vi "Get Data.vi"(8 "error in":errorcluster, 11 "nPAS in":refnum<class "nPAS.lvclass">) -> (0 "error out":errorcluster, 3 "nPAS out":refnum<class "nPAS.lvclass">)   [LabVIEW 2018, in "gPAS Library.lvlib" / "nPAS.lvclass"]
doc: "Here you will do all of your acquisition. The acquisition is going to be implementation dependent, but at the bare minimum the class which inherits the PAS will have to retrieve the speaker signal(s). The data that is acquired in this cycle will be piped to the <b>Analyze Data</b> VI in the next cycle."
uses:
  nPAS.lvclass
  C:/Program Files (x86)/National Instruments/LabVIEW 2018/vi.lib/MSR Consulting, LLC/General Reuse/Instrument/Instrument.lvclass
  <vilib>/MSR Consulting, LLC/General Reuse/PAS/Data/Main/PAS Data.lvclass
  C:/Program Files (x86)/National Instruments/LabVIEW 2018/vi.lib/MSR Consulting, LLC/General Reuse/Data/Data.lvclass
  <vilib>/MSR Consulting, LLC/General Reuse/Instrument/Instrument.lvclass/Instrument.ctl
  <vilib>/MSR Consulting, LLC/General Reuse/PAS/Data/Cell/PAS Cell Data.lvclass/PAS Cell Data.ctl
  <vilib>/MSR Consulting, LLC/General Reuse/Instrument/Read Data.vi
  <vilib>/MSR Consulting, LLC/General Reuse/PAS/Data/Cell/Write lRMS.vi
  <vilib>/MSR Consulting, LLC/General Reuse/Instrument/Write Data.vi
  <vilib>/MSR Consulting, LLC/General Reuse/Instrument/Read Log Session.vi
  <vilib>/MSR Consulting, LLC/General Reuse/PAS/Data/Cell/PAS Cell Data.lvclass
  <vilib>/Utility/error.llb/Error Cluster From Error Code.vi
  <vilib>/rvi/errors/niLvFpgaAdjustHostInterfaceError.vi
  <vilib>/MSR Consulting, LLC/General Reuse/PAS/Data/Main/Read CellData.vi
  <vilib>/MSR Consulting, LLC/General Reuse/Data/Write measTime.vi
  <vilib>/MSR Consulting, LLC/General Reuse/PAS/Data/Cell/Write timeData.vi
  <vilib>/MSR Consulting, LLC/General Reuse/PAS/Data/Cell/Write lasDiodeData.vi
  <vilib>/MSR Consulting, LLC/General Reuse/PAS/Data/Main/Write CellData.vi
  <vilib>/rvi/interface/nirviMethod/nirviMethod.xnode
  FPGA Ref.ctl
  FPGA Bitfiles/server.lvbitx
  <vilib>/rvi/interface/nirviReadWriteControl/nirviReadWriteControl.xnode
  <vilib>/MSR Consulting, LLC/General Reuse/Data/Data.lvclass
  <vilib>/MSR Consulting, LLC/General Reuse/Session APIs/_Session Fwk/Session - Root.lvclass
  <vilib>/MSR Consulting, LLC/General Reuse/Session APIs/Session Log/System Log.lvclass
  <vilib>/FPGAPlugInAG/cRIO-9081/niLvFpga_ReadFifo_cRIO-9081.vi
  <vilib>/rvi/errors/niLvFpgaMergeErrorWithErrorCode.vi
  NiFpgaLv.dll
panel:
  out "Elements Remaining":u32
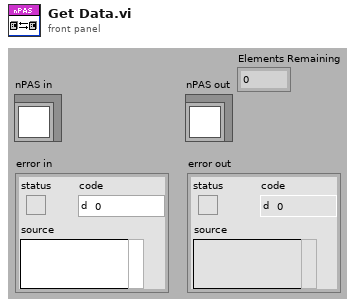
[diagram p1: front panel]
types:
  T1 = typedef "FPGA Ref.ctl" = refnum<k20>
  T2 = typedef "Session - Root.lvclass/Session Handle.ctl" = refnum<data-value>
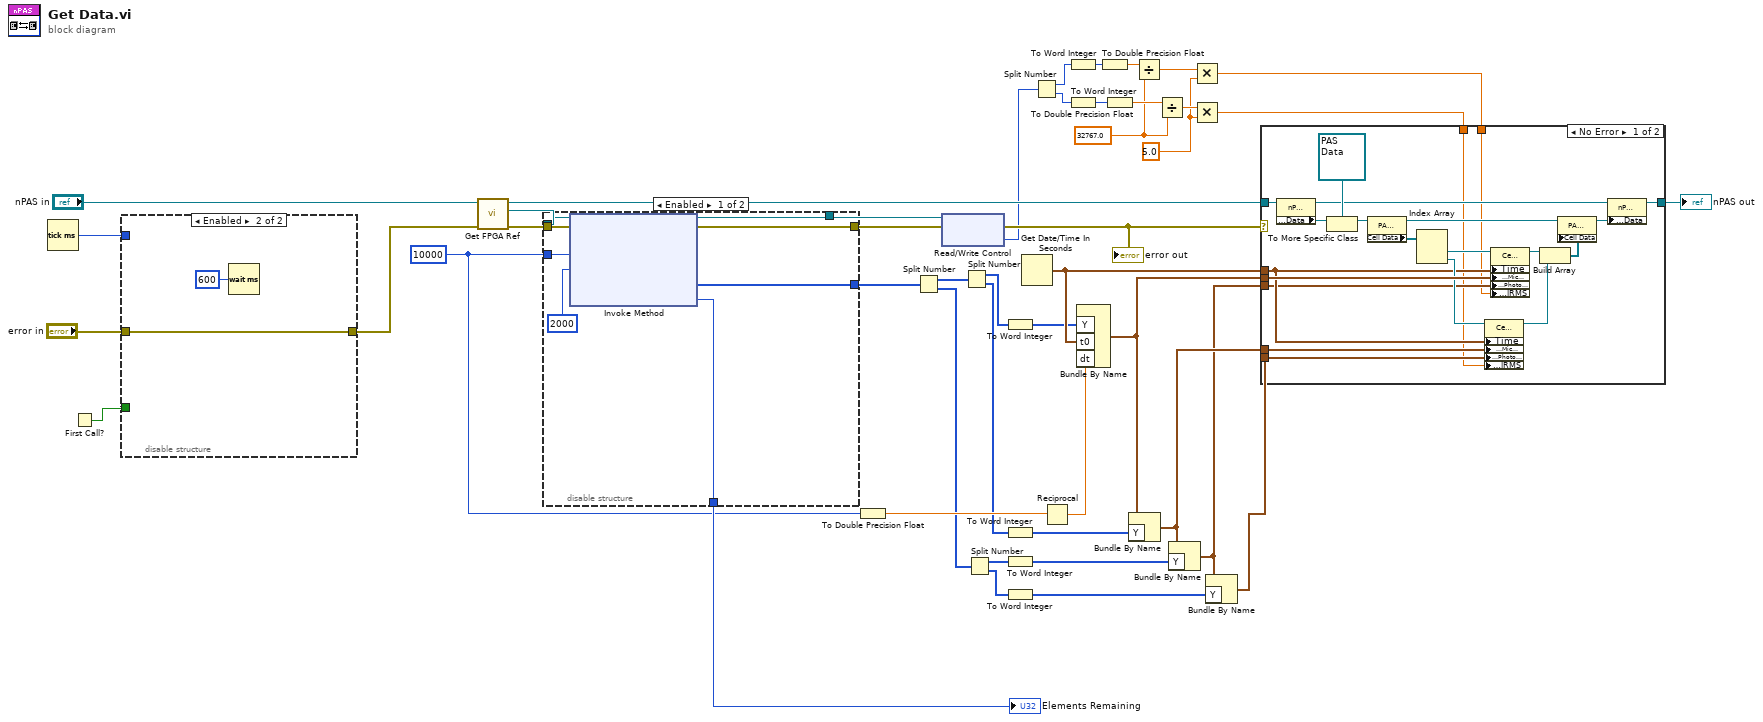
[diagram p0: block diagram]
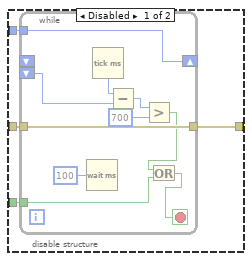
[diagram p2: hidden frame]
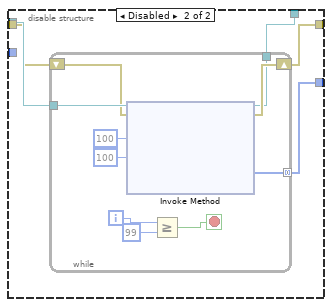
[diagram p3: hidden frame]
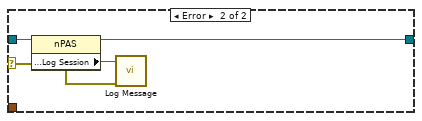
[diagram p4: hidden frame]
diagram:
  w7 = 5.0 ("y")
  w10 = 32767.0
  w42 = u32 10000 ("Number of Elements")
  n1 = Tick Count (ms)() -> (millisecond timer value=w2:u32)
  n2 = First Call?() -> (First Call?: T/F=w1:bool)
  n3 = disable-structure shown="Enabled" {
    disable-tunnel: "error in" -> [w49 w60]
    disable-tunnel: [w48 w60] -> w3
    disable-tunnel: w2 -> [w47 _]
    disable-tunnel: w1 -> [w46 _]
    frame Disabled {
      n4 = while {
        tunnel: w49 -> [w58]
        tunnel: [w58] -> w48
        tunnel: w47 -> [w57]
        shift-right: [w57] -> _
        shift-left: _ -> [_]
        shift-left: _ -> [w55]
        tunnel: w46 -> [w51]
        stop <- w50 stop-if-true
        n5 = Wait (ms)(milliseconds to wait=u32 100) -> ()  [unwired: 1 out]
        n6 = Tick Count (ms)() -> (millisecond timer value=w56:u32)
        n7 = Subtract(x=w56, y=w55) -> (x-y=w54:u32)
        n8 = Greater?(x=w54, y=u32 700) -> (0:w52:bool)
        n9 = Or(x=w52, y=w51) -> (x .or. y?=w50:bool)
      }
    }
    frame Enabled {
      n10 = Wait (ms)(milliseconds to wait=u32 600) -> ()  [unwired: 1 out]
    }
  }
  n11 = call "Get FPGA Ref.vi"("error in"=w3, "nPAS in"="nPAS in") -> ("error out"=w39:errorcluster, "FPGA Ref"=w40:T1, "nPAS out"=w41:refnum<class "nPAS.lvclass">)  [unwired: 7 in]
  n12 = disable-structure shown="Enabled" {
    disable-tunnel: [w69 _] -> w43
    disable-tunnel: w42 -> [w68 _]
    disable-tunnel: w40 -> [w67 w74]
    disable-tunnel: w39 -> [w66 w72]
    disable-tunnel: [w64 w73] -> w38
    disable-tunnel: [w63 w70] -> w36
    disable-tunnel: [w62 w71] -> w35
    frame Enabled {
      n13 = xnode "Invoke Method"("FPGA VI Reference In"=w67, "error in"=w66, "Number of Elements"=w68, "Timeout (ms)"=2000) -> ("FPGA VI Reference Out"=w63:T1, "error out"=w62:errorcluster, "Data"=w64:u64[], "Elements Remaining"=w69:u32)
    }
    frame Disabled {
      n14 = while {
        tunnel: w74 -> [w84]
        tunnel: [w81] -> w73 mode=concatenating
        shift-right: [w76] -> w71
        shift-left: w72 -> [w77]
        tunnel: [w75] -> w70
        i -> [w80]
        stop <- w78 stop-if-true
        n15 = xnode "Invoke Method"("FPGA VI Reference In"=w84, "error in"=w77, "Number of Elements"=u32 100, "Timeout (ms)"=100) -> ("FPGA VI Reference Out"=w75:T1, "error out"=w76:errorcluster, "Data"=w81:u64[])  [unwired: 1 out]
        n16 = Greater Or Equal?(x=w80, y=99) -> (x >= y?=w78:bool)
      }
    }
  }
  "Elements Remaining" <- w43
  n17 = To Double Precision Float(number=w42) -> (double precision float=w37:dbl)
  n18 = Split Number(x=w38) -> (hi(x)=w34:u32[], lo(x)=w33:u32[])
  n19 = xnode "Read/Write Control"("FPGA VI Reference In"=w36, "error in"=w35) -> ("error out"=w18:errorcluster, "pas lrms"=w17:u32)  [unwired: 1 out]
  "error out" <- w18
  n20 = Split Number(x=w34) -> (hi(x)=w26:u16[], lo(x)=w25:u16[])
  n21 = Split Number(x=w33) -> (hi(x)=w24:u16[], lo(x)=w23:u16[])
  n22 = To Word Integer(number=w26) -> (16bit integer=w19:i16[])
  n23 = To Word Integer(number=w25) -> (16bit integer=w20:i16[])
  n24 = To Word Integer(number=w24) -> (16bit integer=w22:i16[])
  n25 = To Word Integer(number=w23) -> (16bit integer=w21:i16[])
  n26 = Get Date/Time In Seconds() -> (seconds since 1Jan1904=w31:timestamp)
  n27 = Split Number(x=w17) -> (hi(x)=w16:u16, lo(x)=w15:u16)
  n28 = Reciprocal(x=w37) -> (1/x=w32:dbl)
  n29 = To Word Integer(number=w16) -> (16bit integer=w13:i16)
  n30 = To Word Integer(number=w15) -> (16bit integer=w12:i16)
  n31 = Bundle By Name("Y"=w19, "t0"=w31, "dt"=w32) -> (w30:waveform(i16))  [unwired: 1 in]
  n32 = To Double Precision Float(number=w13) -> (double precision float=w14:dbl)
  n33 = To Double Precision Float(number=w12) -> (double precision float=w11:dbl)
  n34 = Bundle By Name(cluster=w30, "Y"=w20) -> (w29:waveform(i16))
  n35 = Divide(x=w14, y=w10) -> (x/y=w8:dbl)
  n36 = Divide(x=w11, y=w10) -> (x/y=w9:dbl)
  n37 = Bundle By Name(cluster=w29, "Y"=w22) -> (w28:waveform(i16))
  n38 = Multiply(x=w8, y=w7) -> (x*y=w6:dbl)
  n39 = Multiply(x=w9, y=w7) -> (x*y=w5:dbl)
  n40 = Bundle By Name(cluster=w28, "Y"=w21) -> (w27:waveform(i16))
  n41 = case shown="No Error" w18 {
    selector: w18 -> [_ w107]
    tunnel: w41 -> [w105 w109]
    tunnel: w30 -> [w99 _]
    tunnel: [w93 w106] -> w45
    tunnel: w31 -> [w91 _]
    tunnel: w29 -> [w90 _]
    tunnel: w28 -> [w89 _]
    tunnel: w27 -> [w87 _]
    tunnel: w6 -> [w86 _]
    tunnel: w5 -> [w85 _]
    frame No Error {
      n42 = property class="nPAS"(reference=w105) -> (reference out=w95:refnum<class "nPAS.lvclass">, "Accessors:Data"=w103:refnum<class "Data.lvclass">)  [unwired: 1 in, 1 out]
      n43 = To More Specific Class(target class=refnum<class "PAS Data.lvclass"> refnum ("PAS Library.lvlib:PAS Data"), reference=w103) -> (specific class reference=w101:refnum<class "PAS Data.lvclass">)  [unwired: 1 in, 1 out]
      n44 = property class="PAS Data"(reference=w101) -> (reference out=w98:refnum<class "PAS Data.lvclass">, "Cell Data"=w100:refnum<class "PAS Cell Data.lvclass">[])  [unwired: 1 in, 1 out]
      n45 = Index Array(array=w100) -> (element #1=w104:refnum<class "PAS Cell Data.lvclass">, element #2=w92:refnum<class "PAS Cell Data.lvclass">)  [unwired: 2 in]
      n46 = property class="Cell Data"(reference=w92, "Time"=w91, "Accessors:Mic Time"=w90, "Accessors:Photodiode"=w87, "Accessors:lRMS"=w85) -> (reference out=w88:refnum<class "PAS Cell Data.lvclass">)  [unwired: 1 in, 1 out]
      n47 = property class="Cell Data"(reference=w104, "Time"=w91, "Accessors:Mic Time"=w99, "Accessors:Photodiode"=w89, "Accessors:lRMS"=w86) -> (reference out=w97:refnum<class "PAS Cell Data.lvclass">)  [unwired: 1 in, 1 out]
      n48 = Build Array(w97, w88) -> (w96:refnum<class "PAS Cell Data.lvclass">[])
      n49 = property class="PAS Data"(reference=w98, "Cell Data"=w96) -> (reference out=w94:refnum<class "PAS Data.lvclass">)  [unwired: 1 in, 1 out]
      n50 = property class="nPAS"(reference=w95, "Accessors:Data"=w94) -> (reference out=w93:refnum<class "nPAS.lvclass">)  [unwired: 1 in, 1 out]
    }
    frame Error {
      n51 = property class="nPAS"(reference=w109) -> (reference out=w106:refnum<class "nPAS.lvclass">, "Accessors:Log Session"=w108:T2)  [unwired: 1 in, 1 out]
      n52 = call <vilib>:"Log Message.vi"("error in"=w107, "session in"=w108) -> ()  [unwired: 8 in, 2 out]
    }
  }
  "nPAS out" <- w45
